vi "Queue Overflow and Underflow.vi"() -> ()   [LabVIEW 2023]
doc: "Demonstrates queue operations on a queue with a maximum size. If both loops run at the same speed, the queue does not fill up. When the Enqueue Loop runs fast and the Dequeue Loop runs slow, the queue fills up, and the Enqueue Loop must wait for the Dequeue Loop to remove elements. If the Enqueue Loop runs slow and the Dequeue Loop runs fast, the queue is emptied and the Dequeue Loop must wait for the Enqueue Loop to insert data."
panel:
  in  "Dequeue Speed":u16(ring)=1 items=["Fast (100 ms)", "Slow (500 ms)"]
  in  "Enqueue Speed":u16(ring)=1 items=["Fast (100 ms)", "Slow (500 ms)"]
  out "Dequeued Element":dbl(graph)
  out "Enqueued Element":dbl(graph)
  out "Elements in Queue":i32(slide) scale=0.0..50.0
  in  "Stop":bool
  # "Overview: Demonstrates how using different rates to enqueue and dequeue data with the Queue functions can lead to potential overflow or underflow situations.\nInstructions:\n1. Run the VI.\n2. Note that when the Enqueue Speed equals the Dequeue Speed, the Elements in Queue value remains constant.\n3. Set the Enqueue Speed to Fast. Note that once the queue fills up, the Enqueue Loop must wait to enqueue more elements.\n4. Set the Enqueue Speed back to Slow, and the Dequeue Speed to Fast. Note that once the queue empties, the Dequeue Loop must wait to dequeue more elements.\n5. Click Stop to stop the VI."
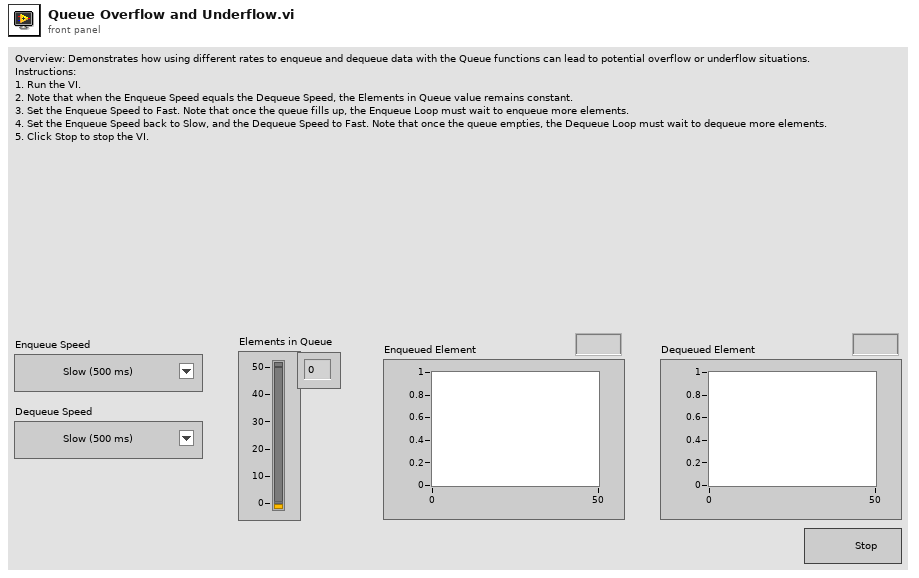
[diagram p1: front panel]
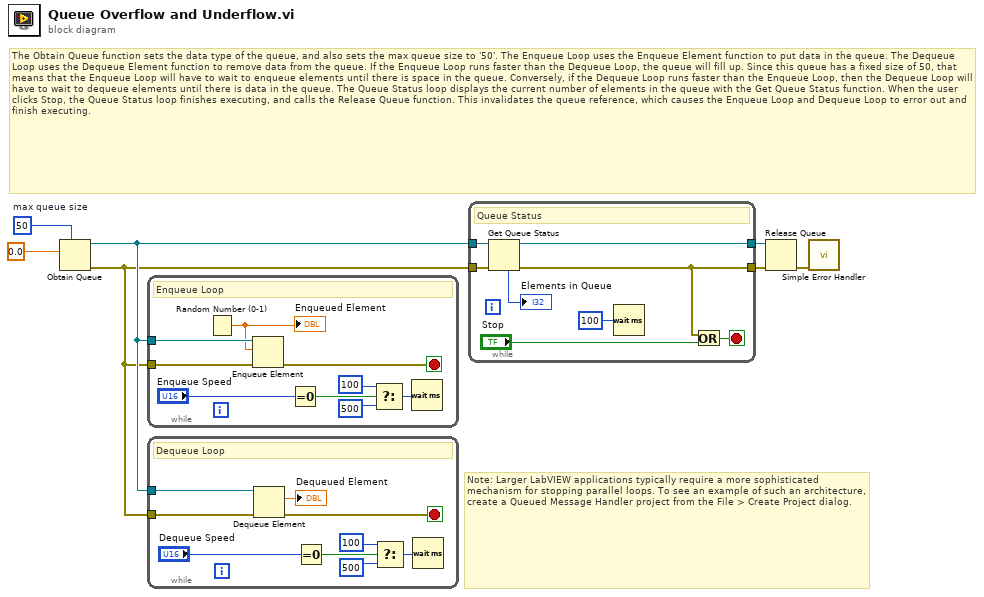
[diagram p0: block diagram]
diagram:
  w1 = 50  # max queue size
  # "Note: Larger LabVIEW applications typically require a more sophisticated mechanism for stopping parallel loops. To see an example of such an architecture, create a Queued Message Handler project from the File > Create Project dialog."
  # "The Obtain Queue function sets the data type of the queue, and also sets the max queue size to '50'. The Enqueue Loop uses the Enqueue Element function to put data in the queue. The Dequeue Loop uses the Dequeue Element function to remove data from the queue. If the Enqueue Loop runs faster than the Dequeue Loop, the queue will fill up. Since this queue has a fixed size of 50, that means that the Enqueue Loop will have to wait to enqueue elements until there is space in the queue. Conversely, if the Dequeue Loop runs faster than the Enqueue Loop, then the Dequeue Loop will have to wait to dequeue elements until there is data in the queue. The Queue Status loop displays the current number of elements in the queue with the Get Queue Status function. When the user clicks Stop, the Queue Status loop finishes executing, and calls the Release Queue function. This invalidates the queue reference, which causes the Enqueue Loop and Dequeue Loop to error out and finish executing."
  n1 = Obtain Queue(max queue size (-1, unlimited)=w1, element data type=0.0) -> (queue out=w7:refnum<queue>, error out=w6:errorcluster)  [unwired: 3 in, 1 out]
  n2 = while {
    tunnel: w7 -> [w16]
    tunnel: w6 -> [w12]
    stop <- w11 stop-if-true
    # "Enqueue Loop"
    n3 = Random Number (0-1)() -> (number: 0 to 1=w10:dbl)
    "Enqueued Element" <- w10
    n4 = Enqueue Element(queue=w16, element=w10, error in (no error)=w12) -> (error out=w11:errorcluster)  [unwired: 3 out]
    n5 = Equal To 0?(x="Enqueue Speed") -> (x = 0?=w8:bool)
    n6 = Select(t=u32 100, s=w8, f=u32 500) -> (s? t:f=w13:u32)
    n7 = Wait (ms)(milliseconds to wait=w13) -> ()  [unwired: 1 out]
  }
  n8 = while {
    tunnel: w7 -> [w25]
    tunnel: w6 -> [w21]
    stop <- w20 stop-if-true
    # "Dequeue Loop"
    n9 = Dequeue Element(queue=w25, error in (no error)=w21) -> (element=→"Dequeued Element":dbl, error out=w20:errorcluster)  [unwired: 3 out]
    n10 = Equal To 0?(x="Dequeue Speed") -> (x = 0?=w17:bool)
    n11 = Select(t=u32 100, s=w17, f=u32 500) -> (s? t:f=w22:u32)
    n12 = Wait (ms)(milliseconds to wait=w22) -> ()  [unwired: 1 out]
  }
  n13 = while {
    tunnel: w7 -> [w33]
    tunnel: [w27] -> w5
    tunnel: w6 -> [w29]
    tunnel: [w28] -> w4
    stop <- w31 stop-if-true
    # "Queue Status"
    n14 = Get Queue Status(queue=w33, error in (no error)=w29) -> (queue out=w28:refnum<queue>, error out=w27:errorcluster, # elements in queue=→"Elements in Queue":i32)  [unwired: 6 out]
    n15 = Wait (ms)(milliseconds to wait=u32 100) -> ()  [unwired: 1 out]
    n16 = Or(x=w27, y="Stop") -> (x .or. y?=w31:bool)
  }
  n17 = Release Queue(queue=w4, error in (no error)=w5) -> (error out=w3:errorcluster)  [unwired: 3 out]
  n18 = call <vilib>:"Simple Error Handler.vi"("error in (no error)"=w3) -> ()  [unwired: 1 in, 8 out]
